vi "Overlay.vi"(8 "error in (no error)":errorcluster, 10 "Image In":T1, 11 "Static Text Overlay In":refnum<class "Static Text Overlay.lvclass">) -> (0 "error out":errorcluster, 2 "Image out":T1, 3 "Static Text Overlay Out":refnum<class "Static Text Overlay.lvclass">)   [LabVIEW 2020, in "Static Text Overlay.lvclass"]
uses:
  Static Text Overlay.lvclass
  C:/POLARIS Programme/POLARIS-AS-3-Cams/Submodules/HIJ Vision/Analyze/Results and Overlays/Results Base/Analyze Results Base.lvclass
  C:/POLARIS Programme/POLARIS-AS-3-Cams/Submodules/HIJ Vision/Analyze/Results and Overlays/Static Overlay/Static Overlay.lvclass
  <vilib>/vision/Image Controls.llb/IMAQ Image.ctl
  Results Base/Analyze Results Base.lvclass/Analyze Results Base.ctl
  Static Overlay/Static Overlay.lvclass/Static Overlay.ctl
  Static Text Overlay.lvclass/Static Text Overlay.ctl
  Results Base/Read Font, Size & Style.vi
  Static Overlay/Read Static Position.vi
  Results Base/Read Overlay colors.vi
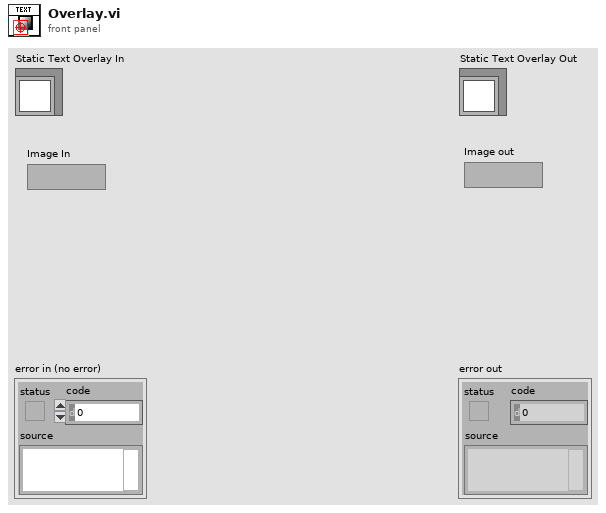
[diagram p1: front panel]
types:
  T1 = typedef "IMAQ Image.ctl" = refnum<image>
  T2 = cluster{"Desired Font (Application)":enum16{"User-specified Font", "Application Font", "System Font", "Dialog Font"}, "[User-specified Font]":cluster{"Font Name":string, "Size":i16, "Strikeout?":bool, "Italic?":bool, "Underline?":bool, "Outline?":bool, "Shadow?":bool, "Bold?":bool, "Rotation Angle":dbl}, "Horizontal Alignment":i16, "Vertical Alignment":i16}
  T3 = typedef "Static Overlay.lvclass/Static Position.ctl" = enum16{"Top Left", "Top Center", "Top Right", "Center", "Bottom Left", "Bottom Center", "Bottom Right"}
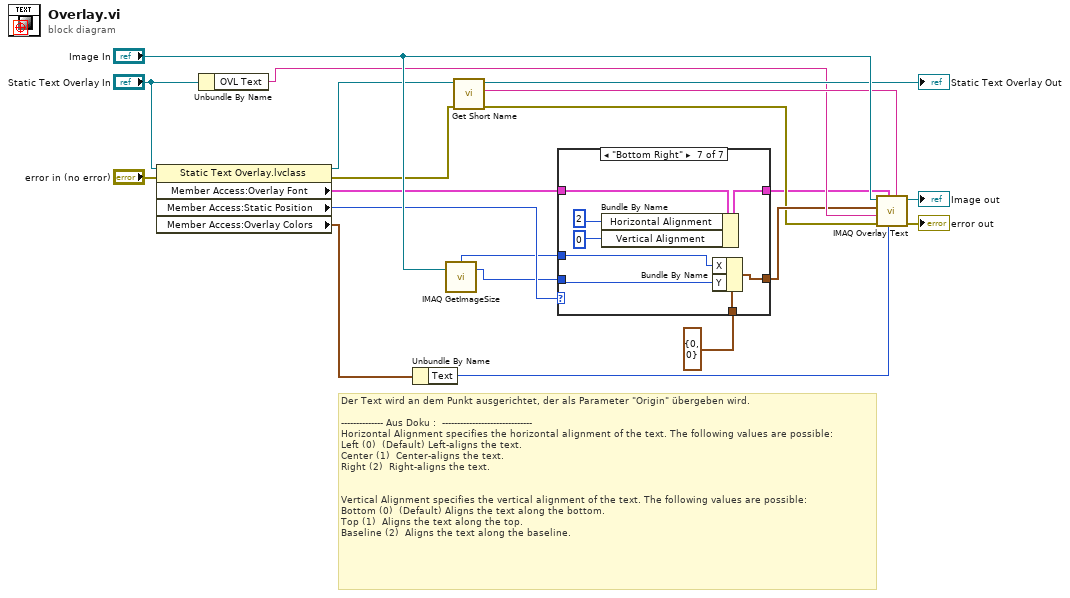
[diagram p0: block diagram]
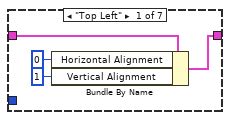
[diagram p2: hidden frame]
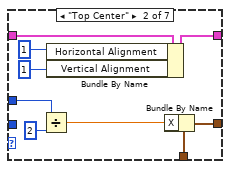
[diagram p3: hidden frame]
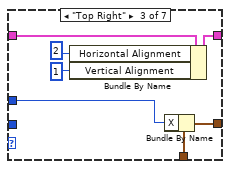
[diagram p4: hidden frame]
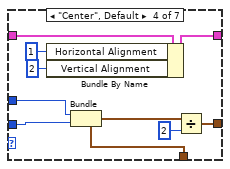
[diagram p5: hidden frame]
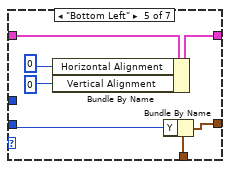
[diagram p6: hidden frame]
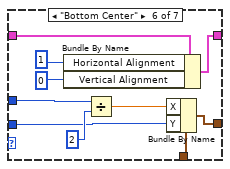
[diagram p7: hidden frame]
diagram:
  # "Der Text wird an dem Punkt ausgerichtet, der als Parameter \"Origin\" übergeben wird.\n\n-------------- Aus Doku :  ------------------------------\nHorizontal Alignment specifies the horizontal alignment of the text. The following values are possible:\nLeft (0) \t(Default) Left-aligns the text.\nCenter (1) \tCenter-aligns the text.\nRight (2) \tRight-aligns the text.\n\n\nVertical Alignment specifies the vertical alignment of the text. The following values are possible:\nBottom (0) \t(Default) Aligns the text along the bottom.\nTop (1) \tAligns the text along the top.\nBaseline (2)  Aligns the text along the baseline."
  n1 = property class="Static Text Overlay.lvclass"(reference="Static Text Overlay In", error in="error in (no error)") -> (reference out=w16:refnum<class "Static Text Overlay.lvclass">, error out=w13:errorcluster, "Member Access:Overlay Font"=w2:T2, "Member Access:Static Position"=w12:T3, "Member Access:Overlay Colors"=w10:cluster{"Border":u32, "Text":u32})
  n2 = Unbundle By Name("Static Text Overlay In") -> ("OVL Text"=w11:string)
  n3 = Unbundle By Name(w10) -> ("Text"=w9:u32)
  n4 = call "IMAQ GetImageSize"("Image"="Image In") -> ("Y Resolution"=w4:i32, "X Resolution"=w5:i32)  [unwired: 3 in, 1 out]
  n5 = call-dynamic "Get Short Name.vi"("error in (no error)"=w13, "Analyze Results Base in"=w16) -> ("error out"=w7:errorcluster, "Short Name"=w14:string, "Analyze Results Base out"=→"Static Text Overlay Out":refnum<class "Static Text Overlay.lvclass">)  [unwired: 7 in]
  n6 = case shown="\"Bottom Right\"" w12 {
    tunnel: [_ w33 w35 w46 w51 w61 w69] -> w8
    tunnel: w5 -> [_ w32 w34 w49 _ w59 w68]
    tunnel: w4 -> [_ _ _ w50 w53 w62 w71]
    tunnel: [w21 w28 w39 w44 w54 w63 w72] -> w3
    tunnel: w2 -> [w22 w29 w40 w45 w55 w64 w73]
    tunnel: cluster{"X":i32, "Y":i32} {"X"=0, "Y"=0} ("Origin") -> [_ w25 w36 w41 w52 w60 w70]
    frame "Top Left" {
      n7 = Bundle By Name(cluster=w22, "Horizontal Alignment"=i16 0, "Vertical Alignment"=i16 1) -> (w21:T2)
    }
    frame "Top Center" {
      n8 = Divide(x=w32, y=2) -> (x/y=w30:dbl)
      n9 = Bundle By Name(cluster=w29, "Horizontal Alignment"=i16 1, "Vertical Alignment"=i16 1) -> (w28:T2)
      n10 = Bundle By Name(cluster=w25, "X"=w30) -> (w33:cluster{"X":i32, "Y":i32})
    }
    frame "Top Right" {
      n11 = Bundle By Name(cluster=w40, "Horizontal Alignment"=i16 2 ("Vertical Alignment"), "Vertical Alignment"=i16 1 ("Horizontal Alignment")) -> (w39:T2)
      n12 = Bundle By Name(cluster=w36, "X"=w34) -> (w35:cluster{"X":i32, "Y":i32})
    }
    frame "Center", Default {
      n13 = Bundle By Name(cluster=w45, "Horizontal Alignment"=i16 1, "Vertical Alignment"=i16 2) -> (w44:T2)
      n14 = Bundle(cluster=w41, "X"=w49, "Y"=w50) -> (w48:cluster{"X":i32, "Y":i32})
      n15 = Divide(x=w48, y=2 ("X Resolution")) -> (x/y=w46:cluster{"X":dbl, "Y":dbl})
    }
    frame "Bottom Left" {
      n16 = Bundle By Name(cluster=w55, "Horizontal Alignment"=i16 0 ("Vertical Alignment"), "Vertical Alignment"=i16 0 ("Horizontal Alignment")) -> (w54:T2)
      n17 = Bundle By Name(cluster=w52, "Y"=w53) -> (w51:cluster{"X":i32, "Y":i32})
    }
    frame "Bottom Center" {
      n18 = Bundle By Name(cluster=w64, "Horizontal Alignment"=i16 1 ("Vertical Alignment"), "Vertical Alignment"=i16 0 ("Horizontal Alignment")) -> (w63:T2)
      n19 = Divide(x=w59, y=2) -> (x/y=w58:dbl)
      n20 = Bundle By Name(cluster=w60, "X"=w58, "Y"=w62) -> (w61:cluster{"X":i32, "Y":i32})
    }
    frame "Bottom Right" {
      n21 = Bundle By Name(cluster=w73, "Horizontal Alignment"=i16 2 ("Vertical Alignment"), "Vertical Alignment"=i16 0 ("Horizontal Alignment")) -> (w72:T2)
      n22 = Bundle By Name(cluster=w70, "X"=w68, "Y"=w71) -> (w69:cluster{"X":i32, "Y":i32})
    }
  }
  n23 = call "IMAQ Overlay Text"("Group"=w14, "Text Color (black)"=w9, "Font, Size & Style"=w3, "error in (no error)"=w7, "String"=w11, "Origin"=w8, "Image"="Image In") -> ("error out"=→"error out":errorcluster, "Image Out"=→"Image out":T1)  [unwired: 3 in]
